vi "LogSourceData_TestOverWrite.vi"(0 "LogFilePath":path) -> (15 "String":string)   [LabVIEW 2011]
panel:
  in  "Ligne à ajouter":string
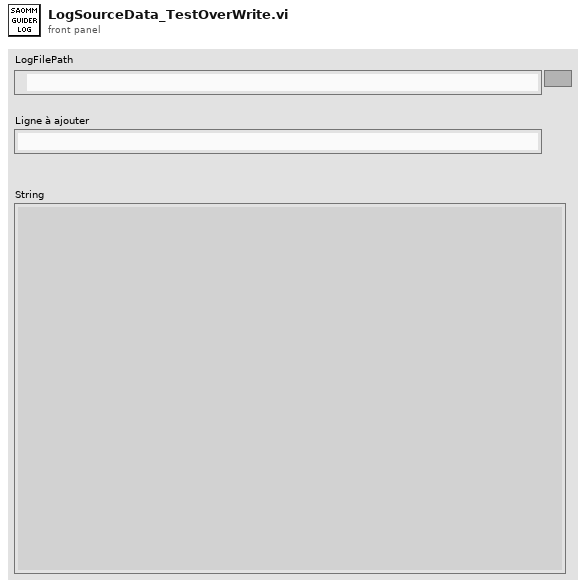
[diagram p1: front panel]
types:
  T1 = enum16{"open", "replace", "create", "open or create", "replace or create", "replace or create with confirmation"}
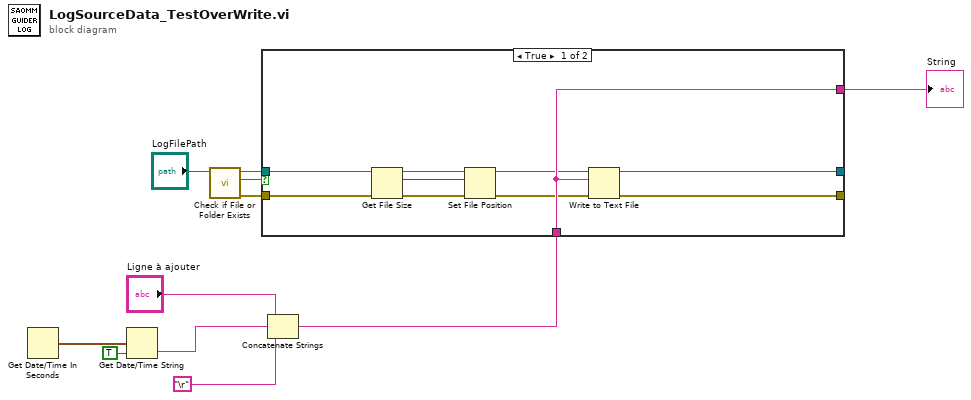
[diagram p0: block diagram]
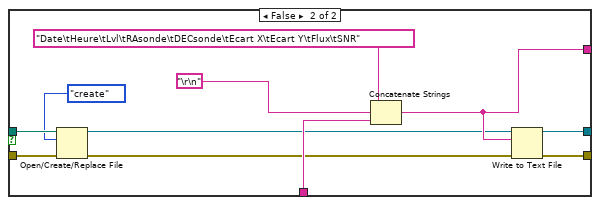
[diagram p2: hidden frame]
diagram:
  n1 = Get Date/Time In Seconds() -> (seconds since 1Jan1904=w6:timestamp)
  n2 = Get Date/Time String(seconds (now)=w6, want seconds? (F)=TRUE) -> (time string=w2:string)  [unwired: 1 in, 1 out]
  n3 = call <vilib>:"Check if File or Folder Exists.vi"("path"="LogFilePath") -> ("error out"=w8:errorcluster, "file or folder exists?"=w10:bool, "dup path"=w9:path)  [unwired: 8 in]
  n4 = Concatenate Strings("Ligne à ajouter", w2, "\r") -> (w3:string)
  n5 = case shown="True" w10 {
    tunnel: w9 -> [w15 w32]
    tunnel: w8 -> [w14 w31]
    tunnel: [w21 w30] -> _
    tunnel: [w20 w29] -> _
    tunnel: w3 -> [w19 w28]
    tunnel: [w19 w27] -> w7
    frame True {
      n6 = Get File Size(file=w15, error in=w14) -> (refnum out=w18:refnum<file>, size (in bytes)=w17:i64, 0:w16:errorcluster)
      n7 = Set File Position(offset (in bytes) (0)=w17, refnum=w18, error in=w16) -> (refnum out=w13:refnum<file>, error out=w12:errorcluster)  [unwired: 1 in]
      n8 = Write to Text File(file (use dialog)=w13, text=w19, error in=w12) -> (refnum out=w21:refnum<file>, error out=w20:errorcluster)  [unwired: 1 in, 1 out]
    }
    frame False {
      n9 = Open/Create/Replace File(file path (use dialog)=w32, error in=w31, operation (0:open)=T1."create") -> (refnum out=w23:refnum<file>, error out=w22:errorcluster)  [unwired: 3 in, 1 out]
      n10 = Concatenate Strings("Date\tHeure\tLvl\tRAsonde\tDECsonde\tEcart X\tEcart Y\tFlux\tSNR", "\r\n", w28) -> (w27:string)
      n11 = Write to Text File(file (use dialog)=w23, text=w27, error in=w22) -> (refnum out=w30:refnum<file>, error out=w29:errorcluster)  [unwired: 1 in, 1 out]
    }
  }
  "String" <- w7
